vi "Detect Array Element Value Change.vi"() -> ()   [LabVIEW 2019]
panel:
  out "element":sgl
  in  "Boolean":bool
  out "id":i32
  in  "ACTR_CMD":sgl[][](array[numeric])
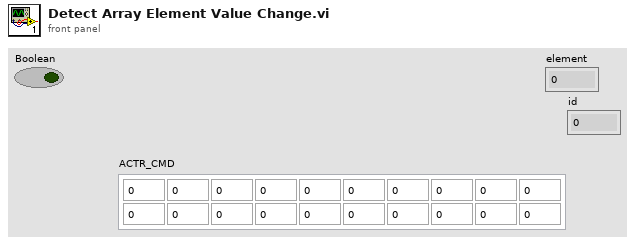
[diagram p1: front panel]
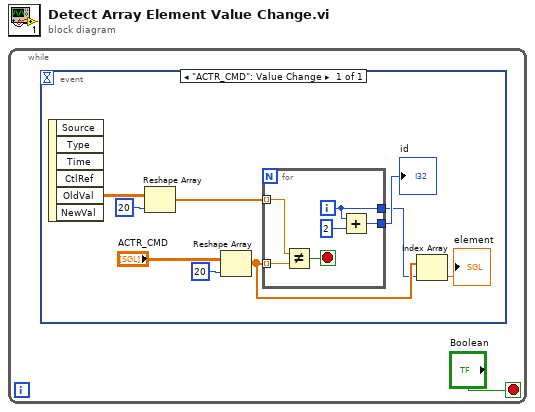
[diagram p0: block diagram]
diagram:
  n1 = while {
    stop <- "Boolean" stop-if-true
    n2 = event shown="[0] \"ACTR_CMD\": Value Change" {
      selector: _ -> [_]
      dyn-events: _ -> [_]
      timeout: _ -> [_]
      event "ACTR_CMD": Value Change {
        n3 = event-data() -> ("OldVal"=w6:sgl[][])  [unwired: 1 in, 5 out]
        n4 = Reshape Array(w6, 20 ("dimension size")) -> (w9:sgl[])
        n5 = Reshape Array("ACTR_CMD", 20 ("dimension size")) -> (w4:sgl[])
        n6 = for {
          tunnel: w9 -> [w16] mode=indexing
          tunnel: w4 -> [w15] mode=indexing
          tunnel: [w12] -> w5
          tunnel: [w11] -> w2
          i -> [w11]
          stop <- w14 stop-if-true
          n7 = Not Equal?(x=w16, y=w15) -> (x != y?=w14:bool)
          n8 = Add(x=w11, y=2) -> (x+y=w12:i32)
        }
        "id" <- w5
        n9 = Index Array(array=w4, index=w2) -> (element=→"element":sgl)
      }
    }
  }
